vi "Nick_newest.vi"() -> ()   [LabVIEW 2017]
uses:
  <vilib>/myRIO/Instrument Drivers/Onboard IO/DIO/typedefs/DIO Reference.ctl
  <vilib>/myRIO/Common/Instrument Driver Framework/Utilities/typedefs/myRIO Generic Hardware Reference.ctl
  <vilib>/myRIO/Common/Instrument Driver Framework/Utilities/typedefs/Hardware Version Enum.ctl
  <vilib>/myRIO/Common/Instrument Driver Framework/Utilities/typedefs/myRIO v1.0 Reference.ctl
  <vilib>/myRIO/Common/Instrument Driver Framework/Utilities/typedefs/Generic FPGA Reference.ctl
  <vilib>/myRIO/Common/Instrument Driver Framework/myRIO v1.0/DIO/typedefs/DIO Channels List.ctl
  <vilib>/myRIO/Common/Instrument Driver Framework/myRIO v1.0/DIO/typedefs/DIO Channels Enum.ctl
  <vilib>/userdefined/High Color/nirio_resource_hc.ctl
  <vilib>/myRIO/Common/Instrument Driver Framework/Utilities/vis/Is FPGA Ref Available.vi
  <vilib>/myRIO/Common/Instrument Driver Framework/myRIO v1.0/DIO/vis/myRIO v1.1 Open DIO.vi
  <vilib>/myRIO/Instrument Drivers/Onboard IO/DIO/vis/Write.vi
  <vilib>/myRIO/Common/Instrument Driver Framework/Utilities/vis/Validate Channels.vi
  <vilib>/myRIO/Common/Instrument Driver Framework/myRIO v1.0/DIO/vis/myRIO v1.0 Reserve DIO.vi
  <vilib>/myRIO/Common/Instrument Driver Framework/myRIO v1.0/Resource Manager/vis/myRIO v1.0 Reserve Channel List.vi
  <vilib>/myRIO/Common/Instrument Driver Framework/myRIO v1.0/DIO/vis/myRIO v1.0 Build MUX Configuration DIO.vi
  <vilib>/myRIO/Common/Instrument Driver Framework/myRIO v1.0/Resource Manager/vis/myRIO v1.0 Reserve Channel.vi
  <vilib>/myRIO/Common/Instrument Driver Framework/myRIO v1.0/Resource Manager/vis/myRIO v1.0 Unreserve Channel.vi
  <vilib>/myRIO/Common/Instrument Driver Framework/myRIO v1.0/Resource Manager/vis/myRIO v1.0 Create Configuration List.vi
  <vilib>/myRIO/Common/Instrument Driver Framework/myRIO v1.0/Resource Manager/vis/myRIO v1.0 Build Mutex Name.vi
  <vilib>/Utility/VariantDataType/GetNumericInfo.vi
  <vilib>/Utility/error.llb/Error Cluster From Error Code.vi
  <vilib>/myRIO/Common/Instrument Driver Framework/myRIO v1.0/myRIO v1.1 Open.vi
  <vilib>/myRIO/Common/Instrument Driver Framework/Utilities/vis/IO Manager.vi
  <vilib>/myRIO/Common/Instrument Driver Framework/Utilities/vis/Configuration Manager.vi
  <vilib>/myRIO/Common/Instrument Driver Framework/myRIO v1.0/Resource Manager/vis/myRIO v1.0 Configure IO.vi
  <vilib>/myRIO/Common/Instrument Driver Framework/myRIO v1.0/myRIO v1.0 Close.vi
  <vilib>/myRIO/Common/Instrument Driver Framework/myRIO v1.0/DIO/vis/myRIO v1.0 Write DIO.vi
  <vilib>/myRIO/Express VI/Onboard IO/DO/DO Express VI.xnode
  <vilib>/myRIO/Instrument Drivers/Onboard IO/DIO/vis/myRIO DIO Open.xnode
  <vilib>/myRIO/Instrument Drivers/Onboard IO/DIO/DIO.lvlib
panel:
  out "Numeric":i32
  out "x+1":i32
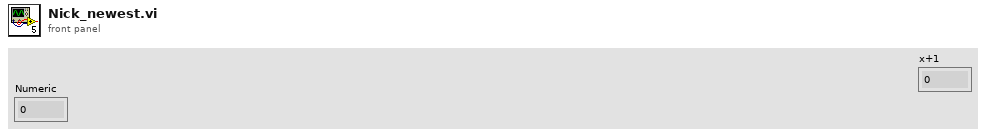
[diagram p1: front panel]
types:
  T1 = typedef "DIO.lvlib/DIO Reference.ctl" = cluster{"myRIO Reference":T2, "DIO Channels List":T6}
  T2 = typedef "myRIO Generic Hardware Reference.ctl" = cluster{"myRIO Model":T3, "myRIO Hardware Reference":T4}
  T3 = typedef "Hardware Version Enum.ctl" = enum16{"Unknown", "myRIO-1900", "myRIO-1950", "roboRIO", "NI ELVIS RIO CM"}
  T4 = typedef "myRIO v1.0 Reference.ctl" = cluster{"Generic FPGA Reference":T5, "Allow multiple opens":bool}
  T5 = typedef "Generic FPGA Reference.ctl" = refnum<k20>
  T6 = typedef "DIO Channels List.ctl" = T7[]
  T7 = typedef "DIO Channels Enum.ctl" = enum16{"Not Connected", "C/DIO0", "C/DIO1", "C/DIO2", "C/DIO3", "C/DIO4", "C/DIO5", "C/DIO6", "C/DIO7", "A/DIO0", "A/DIO1", "A/DIO2", "A/DIO3", "A/DIO4", "A/DIO5", "A/DIO6", "A/DIO7", "A/DIO8", "A/DIO9", "A/DIO10", "A/DIO11", "A/DIO12", "A/DIO13", "A/DIO14", "A/DIO15", "B/DIO0", "B/DIO1", "B/DIO2", "B/DIO3", "B/DIO4", "B/DIO5", "B/DIO6", "B/DIO7", "B/DIO8", "B/DIO9", "B/DIO10", "B/DIO11", "B/DIO12", "B/DIO13", "B/DIO14", "B/DIO15", "LED0", "LED1", "LED2", "LED3", "Button0", "DIO/DIO0", "DIO/DIO1", "DIO/DIO2", "DIO/DIO3", "DIO/DIO4", "DIO/DIO5", "DIO/DIO6", "DIO/DIO7", "DIO/DIO8", "DIO/DIO9", "SPI/CS0", "SPI/CS1", "SPI/CS2", "SPI/CS3", "LED RADIO (Green)", "LED RADIO (Red)", "LED COMM (Green)", "LED COMM (Red)", "LED MODE (Green)", "LED MODE (Red)"}
  T8 = typedef "nirio_resource_hc.ctl" = tag
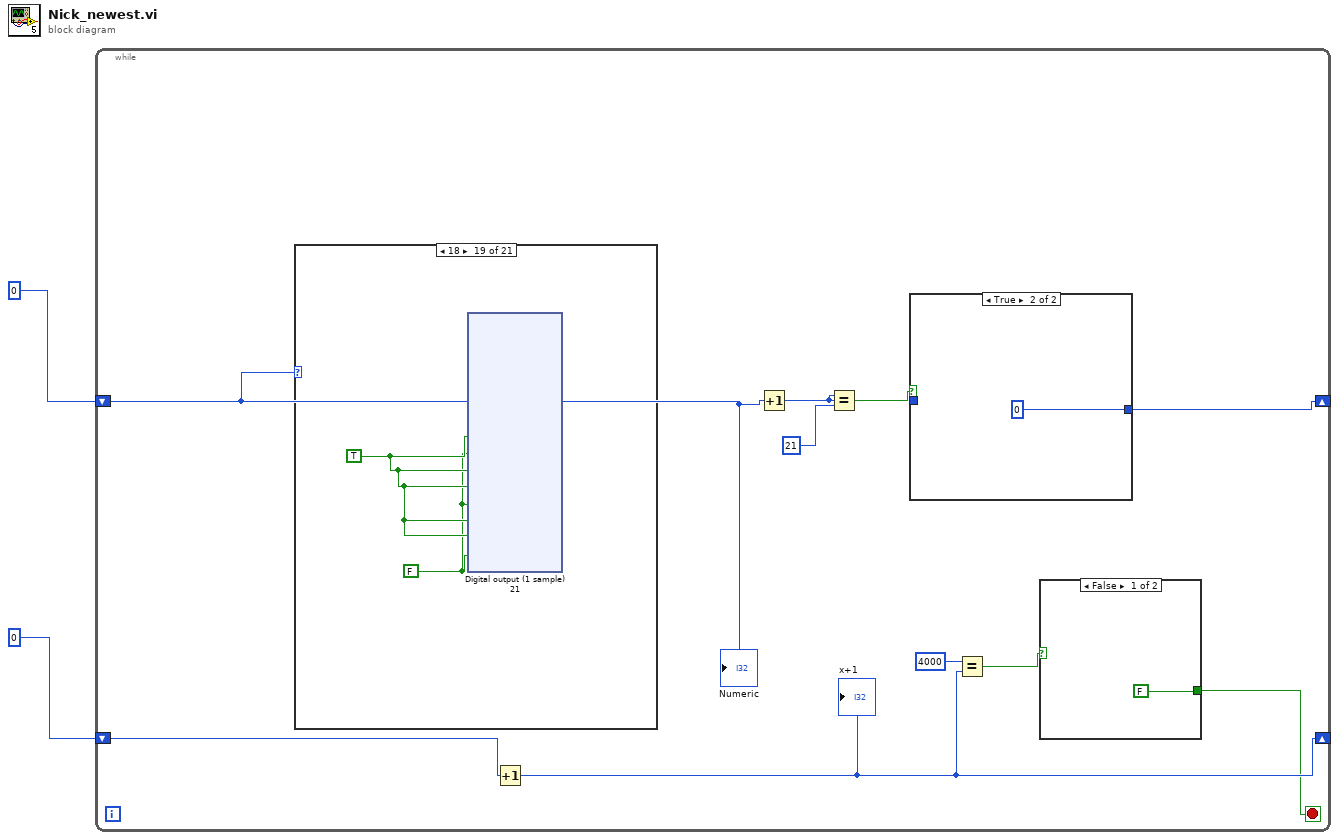
[diagram p0: block diagram]
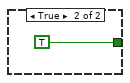
[diagram p2: hidden frame]
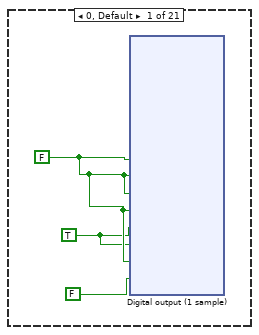
[diagram p4: hidden frame]
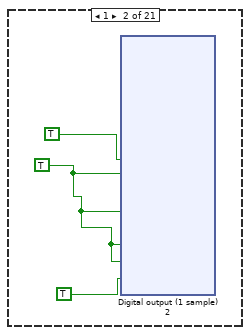
[diagram p5: hidden frame]
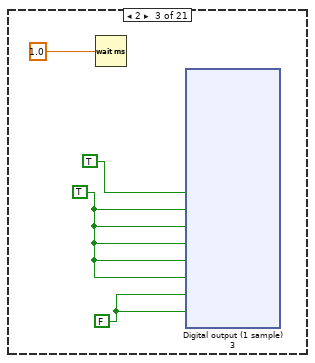
[diagram p6: hidden frame]
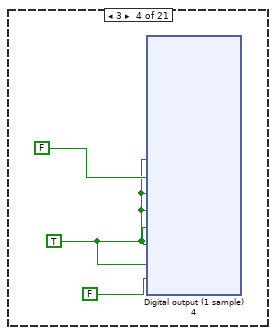
[diagram p7: hidden frame]
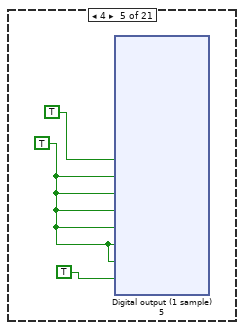
[diagram p8: hidden frame]
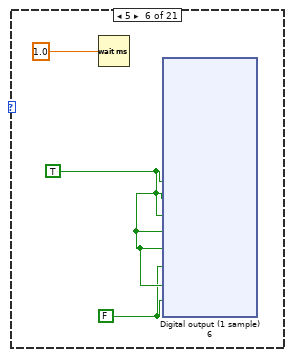
[diagram p9: hidden frame]
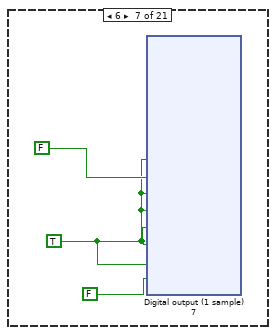
[diagram p10: hidden frame]
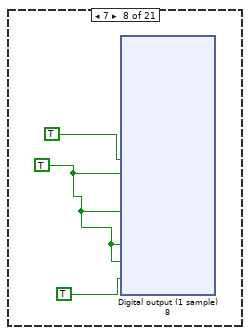
[diagram p11: hidden frame]
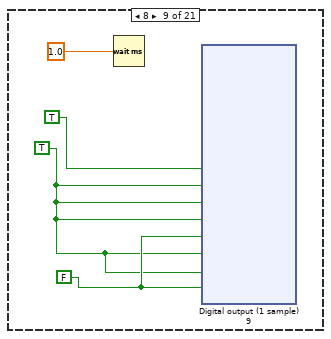
[diagram p12: hidden frame]
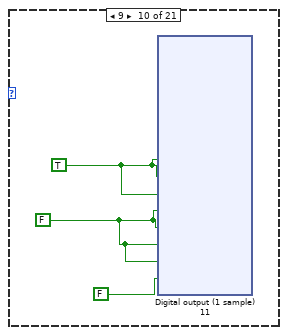
[diagram p13: hidden frame]
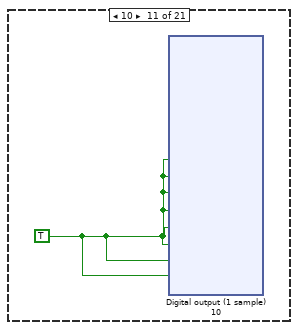
[diagram p14: hidden frame]
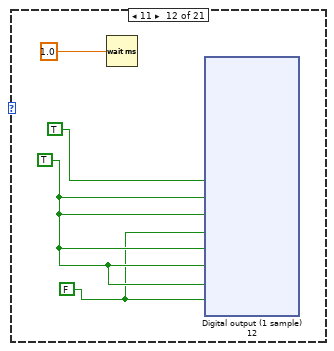
[diagram p15: hidden frame]
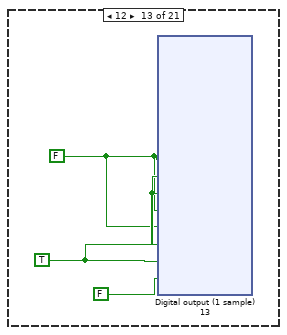
[diagram p16: hidden frame]
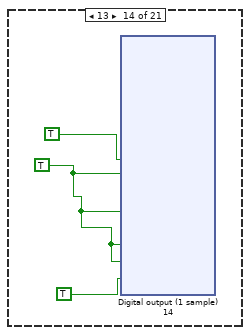
[diagram p17: hidden frame]
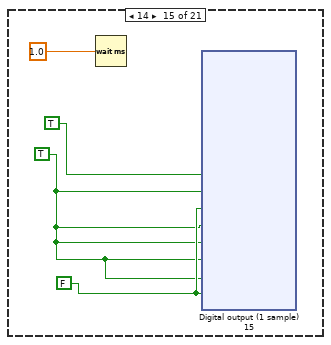
[diagram p18: hidden frame]
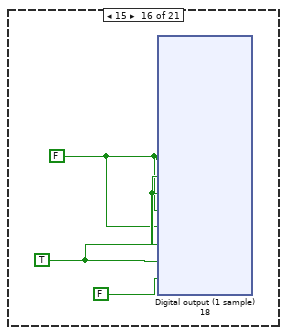
[diagram p19: hidden frame]
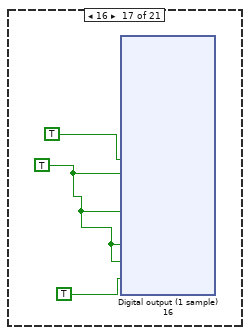
[diagram p20: hidden frame]
diagram:
  n1 = while {
    shift-right: [w9] -> _
    shift-left: 0 -> [w12]
    shift-right: [w6] -> _
    shift-left: 0 -> [w7]
    stop <- w3 stop-if-true
    n2 = case shown="18" w12 {
      frame 0, Default {
        w17 = TRUE
        w18 = FALSE
        n3 = xnode "Digital output (1 sample)"("A/DIO0 (Pin 11)"=w18, "A/DIO1 (Pin 13)"=w18, "A/DIO2 (Pin 15)"=w18, "A/DIO3 (Pin 17)"=w18, "A/DIO4 (Pin 19)"=w17, "A/DIO5 (Pin 21)"=w17, "A/DIO6 (Pin 23)"=w18, "A/DIO7 (Pin 25)"=FALSE) -> ()  [unwired: 1 in, 1 out]
      }
      frame 1 {
        w62 = TRUE
        n4 = xnode "Digital output (1 sample) 2"("A/DIO0 (Pin 11)"=TRUE, "A/DIO1 (Pin 13)"=w62, "A/DIO2 (Pin 15)"=w62, "A/DIO3 (Pin 17)"=w62, "A/DIO4 (Pin 19)"=w62, "A/DIO5 (Pin 21)"=w62, "A/DIO6 (Pin 23)"=w62, "A/DIO7 (Pin 25)"=TRUE) -> ()  [unwired: 1 in, 1 out]
      }
      frame 2 {
        w109 = TRUE
        w108 = FALSE
        n5 = Wait (ms)(milliseconds to wait=1.0) -> ()  [unwired: 1 out]
        n6 = xnode "Digital output (1 sample) 3"("A/DIO0 (Pin 11)"=TRUE, "A/DIO1 (Pin 13)"=w109, "A/DIO2 (Pin 15)"=w109, "A/DIO3 (Pin 17)"=w109, "A/DIO4 (Pin 19)"=w109, "A/DIO5 (Pin 21)"=w109, "A/DIO6 (Pin 23)"=w108, "A/DIO7 (Pin 25)"=w108) -> ()  [unwired: 1 in, 1 out]
      }
      frame 3 {
        w153 = TRUE
        n7 = xnode "Digital output (1 sample) 4"("A/DIO0 (Pin 11)"=w153, "A/DIO1 (Pin 13)"=FALSE, "A/DIO2 (Pin 15)"=w153, "A/DIO3 (Pin 17)"=w153, "A/DIO4 (Pin 19)"=w153, "A/DIO5 (Pin 21)"=w153, "A/DIO6 (Pin 23)"=w153, "A/DIO7 (Pin 25)"=FALSE) -> ()  [unwired: 1 in, 1 out]
      }
      frame 4 {
        w199 = TRUE
        n8 = xnode "Digital output (1 sample) 5"("A/DIO0 (Pin 11)"=TRUE, "A/DIO1 (Pin 13)"=w199, "A/DIO2 (Pin 15)"=w199, "A/DIO3 (Pin 17)"=w199, "A/DIO4 (Pin 19)"=w199, "A/DIO5 (Pin 21)"=w199, "A/DIO6 (Pin 23)"=w199, "A/DIO7 (Pin 25)"=TRUE) -> ()  [unwired: 1 in, 1 out]
      }
      frame 5 {
        w245 = TRUE
        w244 = FALSE
        n9 = Wait (ms)(milliseconds to wait=1.0) -> ()  [unwired: 1 out]
        n10 = xnode "Digital output (1 sample) 6"("A/DIO0 (Pin 11)"=w245, "A/DIO1 (Pin 13)"=w245, "A/DIO2 (Pin 15)"=w245, "A/DIO3 (Pin 17)"=w245, "A/DIO4 (Pin 19)"=w245, "A/DIO5 (Pin 21)"=w244, "A/DIO6 (Pin 23)"=w245, "A/DIO7 (Pin 25)"=w244) -> ()  [unwired: 1 in, 1 out]
      }
      frame 6 {
        w288 = TRUE
        n11 = xnode "Digital output (1 sample) 7"("A/DIO0 (Pin 11)"=w288, "A/DIO1 (Pin 13)"=FALSE, "A/DIO2 (Pin 15)"=w288, "A/DIO3 (Pin 17)"=w288, "A/DIO4 (Pin 19)"=w288, "A/DIO5 (Pin 21)"=w288, "A/DIO6 (Pin 23)"=w288, "A/DIO7 (Pin 25)"=FALSE) -> ()  [unwired: 1 in, 1 out]
      }
      frame 7 {
        w333 = TRUE
        n12 = xnode "Digital output (1 sample) 8"("A/DIO0 (Pin 11)"=TRUE, "A/DIO1 (Pin 13)"=w333, "A/DIO2 (Pin 15)"=w333, "A/DIO3 (Pin 17)"=w333, "A/DIO4 (Pin 19)"=w333, "A/DIO5 (Pin 21)"=w333, "A/DIO6 (Pin 23)"=w333, "A/DIO7 (Pin 25)"=TRUE) -> ()  [unwired: 1 in, 1 out]
      }
      frame 8 {
        w379 = TRUE
        w380 = FALSE
        n13 = Wait (ms)(milliseconds to wait=1.0) -> ()  [unwired: 1 out]
        n14 = xnode "Digital output (1 sample) 9"("A/DIO0 (Pin 11)"=TRUE, "A/DIO1 (Pin 13)"=w379, "A/DIO2 (Pin 15)"=w379, "A/DIO3 (Pin 17)"=w379, "A/DIO4 (Pin 19)"=w380, "A/DIO5 (Pin 21)"=w379, "A/DIO6 (Pin 23)"=w379, "A/DIO7 (Pin 25)"=w380) -> ()  [unwired: 1 in, 1 out]
      }
      frame 9 {
        w424 = FALSE
        w425 = TRUE
        n15 = xnode "Digital output (1 sample) 11"("A/DIO0 (Pin 11)"=w425, "A/DIO1 (Pin 13)"=w425, "A/DIO2 (Pin 15)"=w425, "A/DIO3 (Pin 17)"=w424, "A/DIO4 (Pin 19)"=w424, "A/DIO5 (Pin 21)"=w424, "A/DIO6 (Pin 23)"=w424, "A/DIO7 (Pin 25)"=FALSE) -> ()  [unwired: 1 in, 1 out]
      }
      frame 10 {
        w469 = TRUE
        n16 = xnode "Digital output (1 sample) 10"("A/DIO0 (Pin 11)"=w469, "A/DIO1 (Pin 13)"=w469, "A/DIO2 (Pin 15)"=w469, "A/DIO3 (Pin 17)"=w469, "A/DIO4 (Pin 19)"=w469, "A/DIO5 (Pin 21)"=w469, "A/DIO6 (Pin 23)"=w469, "A/DIO7 (Pin 25)"=w469) -> ()  [unwired: 1 in, 1 out]
      }
      frame 11 {
        w514 = TRUE
        w513 = FALSE
        n17 = Wait (ms)(milliseconds to wait=1.0) -> ()  [unwired: 1 out]
        n18 = xnode "Digital output (1 sample) 12"("A/DIO0 (Pin 11)"=TRUE, "A/DIO1 (Pin 13)"=w514, "A/DIO2 (Pin 15)"=w514, "A/DIO3 (Pin 17)"=w513, "A/DIO4 (Pin 19)"=w514, "A/DIO5 (Pin 21)"=w514, "A/DIO6 (Pin 23)"=w514, "A/DIO7 (Pin 25)"=w513) -> ()  [unwired: 1 in, 1 out]
      }
      frame 12 {
        w558 = FALSE
        w559 = TRUE
        n19 = xnode "Digital output (1 sample) 13"("A/DIO0 (Pin 11)"=w558, "A/DIO1 (Pin 13)"=w559, "A/DIO2 (Pin 15)"=w559, "A/DIO3 (Pin 17)"=w558, "A/DIO4 (Pin 19)"=w558, "A/DIO5 (Pin 21)"=w559, "A/DIO6 (Pin 23)"=w559, "A/DIO7 (Pin 25)"=FALSE) -> ()  [unwired: 1 in, 1 out]
      }
      frame 13 {
        w603 = TRUE
        n20 = xnode "Digital output (1 sample) 14"("A/DIO0 (Pin 11)"=TRUE, "A/DIO1 (Pin 13)"=w603, "A/DIO2 (Pin 15)"=w603, "A/DIO3 (Pin 17)"=w603, "A/DIO4 (Pin 19)"=w603, "A/DIO5 (Pin 21)"=w603, "A/DIO6 (Pin 23)"=w603, "A/DIO7 (Pin 25)"=TRUE) -> ()  [unwired: 1 in, 1 out]
      }
      frame 14 {
        w649 = TRUE
        w650 = FALSE
        n21 = Wait (ms)(milliseconds to wait=1.0) -> ()  [unwired: 1 out]
        n22 = xnode "Digital output (1 sample) 15"("A/DIO0 (Pin 11)"=TRUE, "A/DIO1 (Pin 13)"=w649, "A/DIO2 (Pin 15)"=w650, "A/DIO3 (Pin 17)"=w649, "A/DIO4 (Pin 19)"=w649, "A/DIO5 (Pin 21)"=w649, "A/DIO6 (Pin 23)"=w649, "A/DIO7 (Pin 25)"=w650) -> ()  [unwired: 1 in, 1 out]
      }
      frame 15 {
        w694 = FALSE
        w695 = TRUE
        n23 = xnode "Digital output (1 sample) 18"("A/DIO0 (Pin 11)"=w694, "A/DIO1 (Pin 13)"=w695, "A/DIO2 (Pin 15)"=w695, "A/DIO3 (Pin 17)"=w694, "A/DIO4 (Pin 19)"=w694, "A/DIO5 (Pin 21)"=w695, "A/DIO6 (Pin 23)"=w695, "A/DIO7 (Pin 25)"=FALSE) -> ()  [unwired: 1 in, 1 out]
      }
      frame 16 {
        w739 = TRUE
        n24 = xnode "Digital output (1 sample) 16"("A/DIO0 (Pin 11)"=TRUE, "A/DIO1 (Pin 13)"=w739, "A/DIO2 (Pin 15)"=w739, "A/DIO3 (Pin 17)"=w739, "A/DIO4 (Pin 19)"=w739, "A/DIO5 (Pin 21)"=w739, "A/DIO6 (Pin 23)"=w739, "A/DIO7 (Pin 25)"=TRUE) -> ()  [unwired: 1 in, 1 out]
      }
      frame 17 {
        w786 = TRUE
        w785 = FALSE
        n25 = Wait (ms)(milliseconds to wait=1.0) -> ()  [unwired: 1 out]
        n26 = xnode "Digital output (1 sample) 17"("A/DIO0 (Pin 11)"=TRUE, "A/DIO1 (Pin 13)"=w785, "A/DIO2 (Pin 15)"=w786, "A/DIO3 (Pin 17)"=w786, "A/DIO4 (Pin 19)"=w786, "A/DIO5 (Pin 21)"=w786, "A/DIO6 (Pin 23)"=w786, "A/DIO7 (Pin 25)"=w785) -> ()  [unwired: 1 in, 1 out]
      }
      frame 18 {
        w831 = TRUE
        w830 = FALSE
        n27 = xnode "Digital output (1 sample) 21"("A/DIO0 (Pin 11)"=w831, "A/DIO1 (Pin 13)"=w830, "A/DIO2 (Pin 15)"=w831, "A/DIO3 (Pin 17)"=w831, "A/DIO4 (Pin 19)"=w830, "A/DIO5 (Pin 21)"=w831, "A/DIO6 (Pin 23)"=w831, "A/DIO7 (Pin 25)"=w830) -> ()  [unwired: 1 in, 1 out]
      }
      frame 19 {
        w874 = TRUE
        n28 = xnode "Digital output (1 sample) 19"("A/DIO0 (Pin 11)"=TRUE, "A/DIO1 (Pin 13)"=w874, "A/DIO2 (Pin 15)"=w874, "A/DIO3 (Pin 17)"=w874, "A/DIO4 (Pin 19)"=w874, "A/DIO5 (Pin 21)"=w874, "A/DIO6 (Pin 23)"=w874, "A/DIO7 (Pin 25)"=TRUE) -> ()  [unwired: 1 in, 1 out]
      }
      frame 20 {
        w921 = TRUE
        w920 = FALSE
        n29 = Wait (ms)(milliseconds to wait=1.0) -> ()  [unwired: 1 out]
        n30 = xnode "Digital output (1 sample) 20"("A/DIO0 (Pin 11)"=w920, "A/DIO1 (Pin 13)"=w921, "A/DIO2 (Pin 15)"=w921, "A/DIO3 (Pin 17)"=w921, "A/DIO4 (Pin 19)"=w921, "A/DIO5 (Pin 21)"=w921, "A/DIO6 (Pin 23)"=w921, "A/DIO7 (Pin 25)"=w920) -> ()  [unwired: 1 in, 1 out]
      }
    }
    n31 = Increment(x=w7) -> (x+1=w6:i32)
    "x+1" <- w6
    n32 = Increment(x=w12) -> (x+1=w8:i32)
    n33 = Equal?(x=w8, y=21) -> (x = y?=w10:bool)
    n34 = case shown="True" w10 {
      tunnel: [w15 0] -> w9
      tunnel: w8 -> [w15 _]
      frame False {
      }
      frame True {
      }
    }
    n35 = Equal?(x=4000, y=w6) -> (x = y?=w4:bool)
    n36 = case shown="False" w4 {
      tunnel: [FALSE TRUE] -> w3
      frame False {
      }
      frame True {
      }
    }
    "Numeric" <- w12
  }
